vi "poly_xwav2xy_multi.vi"(7 "XY graph":refnum<vi>, 8 "error in":errorcluster, 10 "relative x? (F)":bool, 11 "xwavs in":T1[](array[typedef])) -> (0 "error out":errorcluster, 1 "xy array out":cluster{"X":dbl[], "Y":dbl[]}[](array[cluster]), 2 "y units":string[](array[string]), 3 "x units":string[](array[string]), 4 "x dimentions":string[](array[string]))   [LabVIEW 2015, in "_xwav_polys.lvlib"]
uses:
  _xwav_polys.lvlib
  xwav.ctl
  <vilib>/Utility/Data Type/NI_Data Type.lvlib
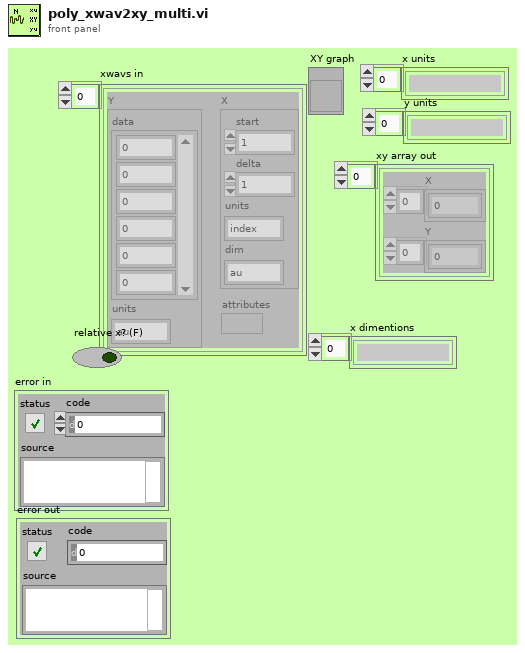
[diagram p1: front panel]
types:
  T1 = typedef "xwav.ctl" = cluster{"attributes":variant, "X":cluster{"start":dbl, "delta":dbl, "units":string, "dim":string}, "Y":cluster{"data":dbl[], "units":string}}
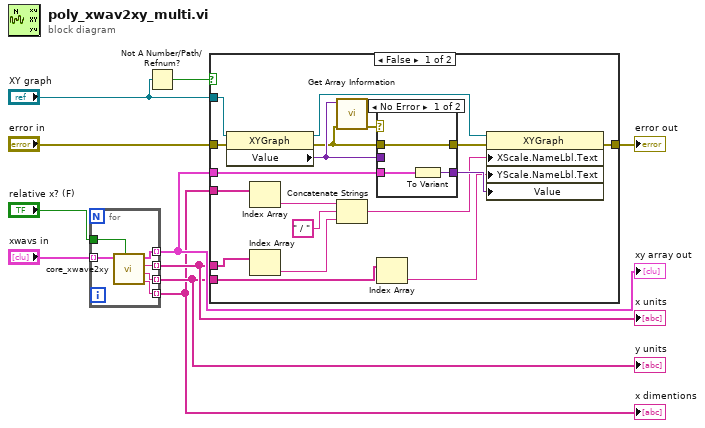
[diagram p0: block diagram]
diagram:
  n1 = for {
    tunnel: "xwavs in" -> [w16] mode=indexing
    tunnel: "relative x? (F)" -> [w15]
    tunnel: [w14] -> w7 mode=indexing
    tunnel: [w13] -> w3 mode=indexing
    tunnel: [w12] -> w2 mode=indexing
    tunnel: [w11] -> w1 mode=indexing
    n2 = call "core_xwave2xy.vi"("relative x? (F)"=w15, "xwave"=w16) -> ("x dimention"=w11:string, "y units"=w12:string, "x units"=w13:string, "xy cluster"=w14:cluster{"X":dbl[], "Y":dbl[]})  [unwired: 6 in]
  }
  "xy array out" <- w7
  "x dimentions" <- w1
  "x units" <- w3
  "y units" <- w2
  n3 = Not A Number/Path/Refnum?(number/path/refnum="XY graph") -> (NaN/Path/Refnum?=w8:bool)
  n4 = case shown="False" w8 {
    tunnel: "XY graph" -> [w34 _]
    tunnel: [w25 w40] -> w6
    tunnel: "error in" -> [w24 w40]
    tunnel: w7 -> [w23 _]
    tunnel: w3 -> [w22 _]
    tunnel: w2 -> [w20 _]
    tunnel: w1 -> [w18 _]
    frame False {
      n5 = property class="XYGraph"(reference=w34, error in=w24) -> (reference out=w33:refnum<vi>, error out=w28:errorcluster, "Value"=w30:variant)
      n6 = Index Array(array=w18) -> (element=w17:string)  [unwired: 1 in]
      n7 = Index Array(array=w22) -> (element=w21:string)  [unwired: 1 in]
      n8 = call <vilib>:"Get Array Information.vi"("error in (no error)"=w28, "Variant"=w30) -> ("error out"=w32:errorcluster)  [unwired: 6 in, 3 out]
      n9 = Concatenate Strings(w17, " / " ("string"), w21) -> (w26:string)
      n10 = case shown="No Error" w32 {
        tunnel: [w37 w38] -> w31
        tunnel: w30 -> [_ w38]
        tunnel: [w36 w39] -> w29
        tunnel: w28 -> [w36 w39]
        tunnel: w23 -> [w35 _]
        frame No Error {
          n11 = To Variant(anything=w35) -> (Variant=w37:variant)
        }
        frame Error {
        }
      }
      n12 = Index Array(array=w20) -> (element=w19:string)  [unwired: 1 in]
      n13 = property class="XYGraph"(reference=w33, error in=w29, "XScale.NameLbl.Text"=w26, "YScale.NameLbl.Text"=w19, "Value"=w31) -> (error out=w25:errorcluster)  [unwired: 1 out]
    }
    frame True {
    }
  }
  "error out" <- w6
